vi "Get JSON API Documentation.vi"(8 "error in (no error)":errorcluster, 11 "Help":refnum<class "Help.lvclass">) -> (0 "error out":errorcluster, 2 "<JSON> API documentation":string, 3 "Help out":refnum<class "Help.lvclass">)   [LabVIEW 2019, in "Help.lvclass"]
uses:
  Help.lvclass
  Help.lvclass/Help.ctl
  ca868cea-1423-40d0-bede-52914c02769a.vi
  47e4b0b2-8925-4823-9c6b-443795284c27.vi
  <vilib>/JDP Science/JSONtext/Variant to JSON Text.vi
  <vilib>/JDP Science/JSONtext/LVClass Serializer/JSONtext LVClass Serializer.lvclass
  <vilib>/JDP Science/JSONtext/JSONtext.lvlib
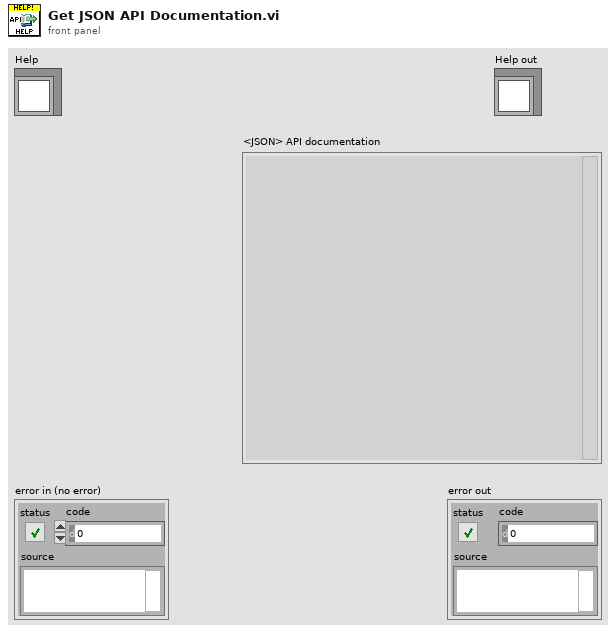
[diagram p1: front panel]
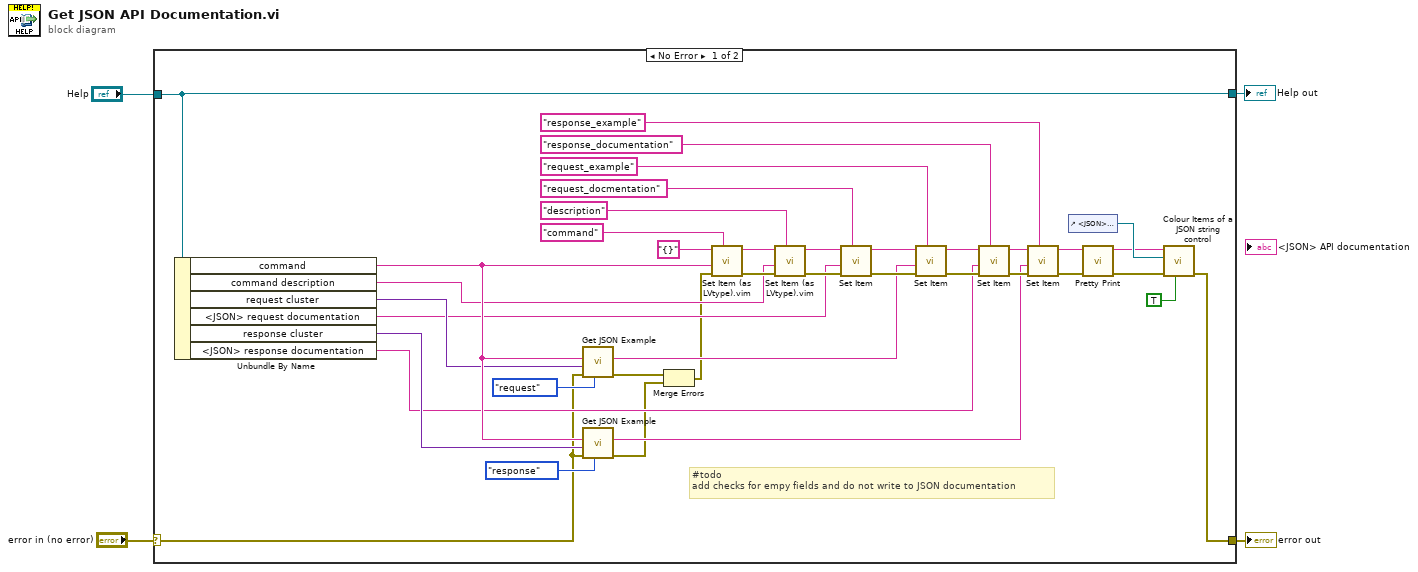
[diagram p0: block diagram]
diagram:
  n1 = case shown="No Error" "error in (no error)" {
    selector: "error in (no error)" -> [w5 w45]
    tunnel: [w27 w45] -> w3
    tunnel: "Help" -> [w11 w44]
    tunnel: [w11 w44] -> w1
    frame No Error {
      # "#todo\nadd checks for empy fields and do not write to JSON documentation"
      n2 = Unbundle By Name(w11) -> ("command"=w15:string, "command description"=w14:string, "request cluster"=w13:variant, "<JSON> request documentation"=w10:string, "response cluster"=w12:variant, "<JSON> response documentation"=w9:string)
      n3 = call "Get JSON Example.vi"("type"=enum16{"request", "response"}."request", "error in (no error)"=w5, "params"=w13, "method"=w15) -> ("error out"=w8:errorcluster, "<JSON>"=w17:string)  [unwired: 6 in]
      n4 = call "Get JSON Example.vi"("type"=enum16{"request", "response"}."response", "error in (no error)"=w5, "params"=w12, "method"=w15) -> ("error out"=w7:errorcluster, "<JSON>"=w16:string)  [unwired: 6 in]
      n5 = Merge Errors(w8, w7) -> (w6:errorcluster)
      n6 = call "Set Item (as LVtype).vim"("$Path or Item Name"="command", "error in (no error)"=w6, "Anything"=w15, "JSON"="{}") -> ("error out"=w23:errorcluster, "<JSON>"=w26:string)  [unwired: 4 in, 1 out]
      n7 = call "Set Item (as LVtype).vim"("$Path or Item Name"="description", "error in (no error)"=w23, "Anything"=w14, "JSON"=w26) -> ("error out"=w37:errorcluster, "<JSON>"=w38:string)  [unwired: 4 in, 1 out]
      n8 = call <vilib>:"Set Item.vi"("$Path or Item Name"="request_docmentation", "error in (no error)"=w37, "JSON to Insert"=w10, "JSON"=w38) -> ("error out"=w32:errorcluster, "<JSON>"=w33:string)  [unwired: 4 in, 1 out]
      n9 = call <vilib>:"Set Item.vi"("$Path or Item Name"="request_example", "error in (no error)"=w32, "JSON to Insert"=w17, "JSON"=w33) -> ("error out"=w30:errorcluster, "<JSON>"=w31:string)  [unwired: 4 in, 1 out]
      n10 = call <vilib>:"Set Item.vi"("$Path or Item Name"="response_documentation", "error in (no error)"=w30, "JSON to Insert"=w9, "JSON"=w31) -> ("error out"=w35:errorcluster, "<JSON>"=w34:string)  [unwired: 4 in, 1 out]
      n11 = call <vilib>:"Set Item.vi"("$Path or Item Name"="response_example", "error in (no error)"=w35, "JSON to Insert"=w16, "JSON"=w34) -> ("error out"=w21:errorcluster, "<JSON>"=w22:string)  [unwired: 4 in, 1 out]
      n12 = control-ref of="<JSON> API documentation"() -> (w43:refnum<vi>)
      n13 = call <vilib>:"Pretty Print.vi"("error in (no error)"=w21, "JSON"=w22) -> ("error out"=w41:errorcluster, "<JSON>"=w20:string)  [unwired: 7 in, 1 out]
      n14 = call <vilib>:"Colour Items of a JSON string control.vi"("Defer Panel Updates"=TRUE, "error in (no error)"=w41, "String Control"=w43, "JSON"=w20) -> ("error out"=w27:errorcluster)  [unwired: 7 in]
    }
    frame Error {
    }
  }
  "error out" <- w3
  "Help out" <- w1
